vi "PSTR-Huet Model.vi"(3 "output control":T1, 4 "data":variant, 5 "X":dbl[](array[numeric]), 6 "a":dbl[](array[numeric])) -> (0 "error out":errorcluster, 1 "f'(X,a)":dbl[][](array[numeric]), 2 "f(X,a)":dbl[](array[numeric]))   [LabVIEW 2015]
doc: "Sum of three Gaussians, plus DC offset."
uses:
  <vilib>/gmath/NumericalOptimization/LM_output select.ctl
  <vilib>/gmath/NI_Gmath.lvlib
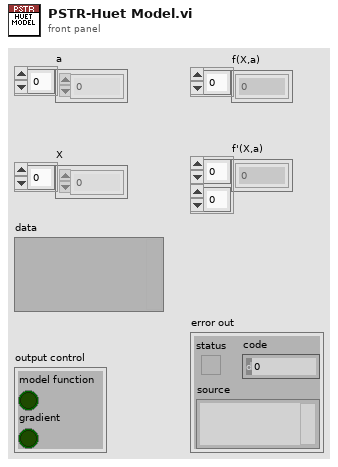
[diagram p1: front panel]
types:
  T1 = typedef "NI_Gmath.lvlib/LM_output select.ctl" = cluster{"model function":bool, "gradient":bool}
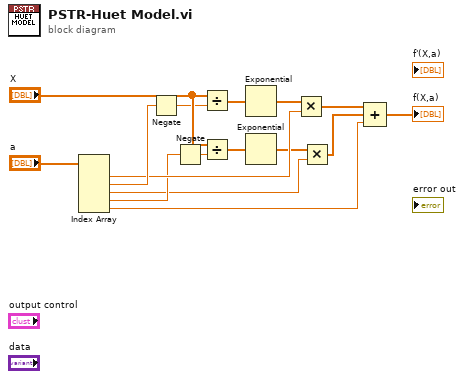
[diagram p0: block diagram]
diagram:
  n1 = Index Array(array="a") -> (element #1=w13:dbl, element #2=w15:dbl, element #3=w10:dbl, element #4=w12:dbl, element #5=w6:dbl)  [unwired: 5 in]
  n2 = Negate(x=w15) -> (-x=w4:dbl)
  n3 = Negate(x=w12) -> (-x=w3:dbl)
  n4 = Divide(x="X", y=w4) -> (x/y=w14:dbl[])
  n5 = Divide(x="X", y=w3) -> (x/y=w9:dbl[])
  n6 = Exponential(1:w14) -> (0:w2:dbl[])
  n7 = Exponential(1:w9) -> (0:w1:dbl[])
  n8 = Multiply(x=w2, y=w13) -> (x*y=w8:dbl[])
  n9 = Multiply(x=w1, y=w10) -> (x*y=w7:dbl[])
  n10 = Compound Arithmetic op=ADD(w8, w7, w6) -> (→"f(X,a)":dbl[])
